vi "CAN Read.vi"(8 "error in (no error)":errorcluster, 9 "TimestampBuffer in":T1, 10 "MessageBuffer in":T2 {"ID" format="%x"; "MSGTYPE" format="%x"; "LEN" format="%x"; "DATA[0]" format="%x"; "DATA[1]" format="%x"; "DATA[2]" format="%x"; "DATA[3]" format="%x"; "DATA[4]" format="%x"; "DATA[5]" format="%x"; "DATA[6]" format="%x"; "DATA[7]" format="%x"}, 11 "Channel":u16) -> (0 "error out":errorcluster, 1 "TimestampBuffer out":T1, 2 "MessageBuffer out":T2 {"ID" format="%x"; "MSGTYPE" format="%x"; "LEN" format="%x"; "DATA[0]" format="%x"; "DATA[1]" format="%x"; "DATA[2]" format="%x"; "DATA[3]" format="%x"; "DATA[4]" format="%x"; "DATA[5]" format="%x"; "DATA[6]" format="%x"; "DATA[7]" format="%x"}, 3 "function return":u32)   [LabVIEW 2020, in "PCANBasic_eX.lvlib"]
doc: "TPCANStatus __stdcall CAN_Read(\n TPCANHandle Channel, \n TPCANMsg* MessageBuffer, \n TPCANTimestamp* TimestampBuffer);"
uses:
  PCANBasic_eX.lvlib
  eX/CTLs/CAN MSG_eX.ctl
  eX/CTLs/CAN Timestamp_eX.ctl
  PCANBasic.dll
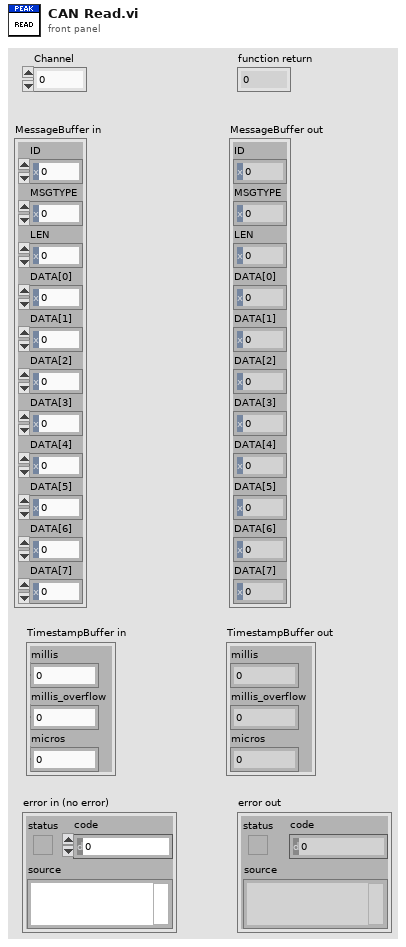
[diagram p1: front panel]
types:
  T1 = typedef "PCANBasic_eX.lvlib/CAN Timestamp_eX.ctl" = cluster{"millis":u32, "millis_overflow":u16, "micros":u16}
  T2 = typedef "PCANBasic_eX.lvlib/CAN MSG_eX.ctl" = cluster{"ID":u32, "MSGTYPE":u8, "LEN":u8, "DATA[0]":u8, "DATA[1]":u8, "DATA[2]":u8, "DATA[3]":u8, "DATA[4]":u8, "DATA[5]":u8, "DATA[6]":u8, "DATA[7]":u8}
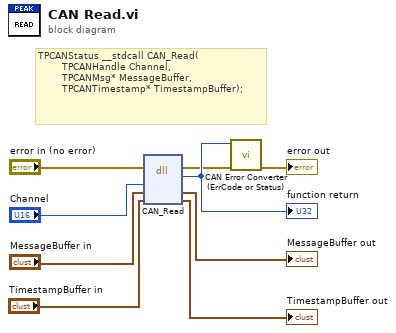
[diagram p0: block diagram]
diagram:
  # "TPCANStatus __stdcall CAN_Read(\n        TPCANHandle Channel, \n        TPCANMsg* MessageBuffer, \n        TPCANTimestamp* TimestampBuffer);"
  n1 = dll-call lib="PCANBasic.*" fn="CAN_Read"(error in="error in (no error)", "Channel"="Channel", "MessageBuffer"="MessageBuffer in", "TimestampBuffer"="TimestampBuffer in") -> (error out=w6:errorcluster, w9:u32, "MessageBuffer"=→"MessageBuffer out":T2, "TimestampBuffer"=→"TimestampBuffer out":T1)  [unwired: 3 in, 1 out]
  "function return" <- w9
  n2 = call "CAN Error Converter (ErrCode or Status).vi"("error in (no error)"=w6, "error code"=w9) -> ("error out"=→"error out":errorcluster)  [unwired: 9 in]
